vi "Mcp2210 Get Spi Config.vi"(6 "error in (no error)":errorcluster, 9 "handle":i32) -> (0 "error out":errorcluster, 2 "SPI Setting Out":T1 {"SPI Mode" items=["Mode 0", "Mode 1", "Mode 2", "Mode 3"]; "Baud Rate" format="%.0p"}, 3 "handle out":i32)   [LabVIEW 2015, in "mcp2210.lvlib"]
doc: "Get the SPI transfer settings for current (VM) configuration or for power-up\ndefault (NVRAM) SPI configuration.\nParameters:\nInputs:\n- void *handle - The pointer to the device handle. Cannot be NULL.\n- unsigned char cfgSelector - current/power-up chip setting selection. Valid values are:\n- MCP2210_VM_CONFIG: designates current chip setting (Volatile\nMemory)\n- MCP2210_NVRAM_CONFIG: designates power-up chip setting (NVRAM)\nOutputs:\n- unsigned int *pbaudRate - transfer speed. Cannot be NULL.\n- unsigned int *pidleCsVal - IDLE chip select value. Cannot be NULL.\nbit31 - - - - bit8 bit0\nx x ... x x CS8 CS7 CS6 CS5 CS4 CS3 CS2 CS1 CS0\n- unsigned int *pactiveCsVal - Active Chip Select Value. Cannot be NULL.\nbit31 - - - - bit8 bit0\nx x ... x x CS8 CS7 CS6 CS5 CS4 CS3 CS2 CS1 CS0\n- unsigned int *pCsToDataDly - Chip Select to Data Delay (quanta of 100 us)\n- 16-bit value => max value is (2^16-1).\n- Cannot be NULL.\n- unsigned int *pdataToCsDly - Last Data Byte to CS (de-asserted) Delay (quanta of 100 us)\n- 16-bit value => max value is (2^16)-1.\n- Cannot be NULL.\n- unsigned int *pdataToDataDly - Delay Between Subsequent Data Bytes (quanta of 100 us)\n- 16-bit value => max value is (2^16)-1.\n- Cannot be NULL.\n- unsigned int *ptxferSize - Bytes to Transfer per SPI Transaction.\n- 16-bit value => max value is (2^16)-1.\n- Cannot be NULL.\n- unsigned char *pspiMd - SPI Mode. Cannot be NULL.\nValid values are:\n- MCP2210_SPI_MODE0\n- MCP2210_SPI_MODE1\n- MCP2210_SPI_MODE2\n- MCP2210_SPI_MODE3\nReturns:\n- 0 for success: E_SUCCESS\n- negative error code: E_ERR_NULL, E_ERR_INVALID_HANDLE_VALUE\nE_ERR_UNKOWN_ERROR, E_ERR_INVALID_PARAMETER\nE_ERR_HID_TIMEOUT, E_ERR_HID_RW_FILEIO\nE_ERR_CMD_ECHO, E_ERR_CMD_FAILED\n\nMCP2210_DLL_UM_API int __stdcall Mcp2210_GetSpiConfig(void *handle, unsigned char cfgSelector, unsigned int *pbaudRate, unsigned int *pidleCsVal,\n unsigned int *pactiveCsVal, unsigned int *pCsToDataDly, unsigned int *pdataToCsDly,\n unsigned int *pdataToDataDly, unsigned int *ptxferSize, unsigned char *pspiMd);"
uses:
  <userlib>/mcp2210/mcp2210.lvlib
  <userlib>/mcp2210/mcp2210_dll_um_x86.dll
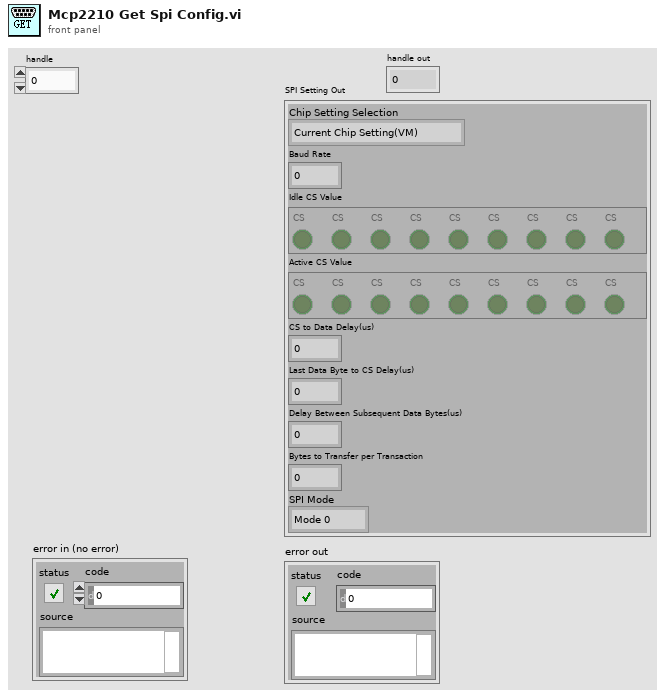
[diagram p1: front panel]
types:
  T1 = cluster{"Chip Setting Selection":enum8{"Current Chip Setting(VM)", "Power-up Chip Setting(NVRAM)"}, "Baud Rate":u32, "Idle CS Value":bool[], "Active CS Value":bool[], "CS to Data Delay(us)":u32, "Last Data Byte to CS Delay(us)":u32, "Delay Between Subsequent Data Bytes(us)":u32, "Bytes to Transfer per Transaction":u32, "SPI Mode":u8}
  T2 = cluster{"cfgSelector":u8, "pbaudRate":u32, "Boolean array":bool[], "Boolean array":bool[], u32, u32, u32, "ptxferSize":u32, u8}
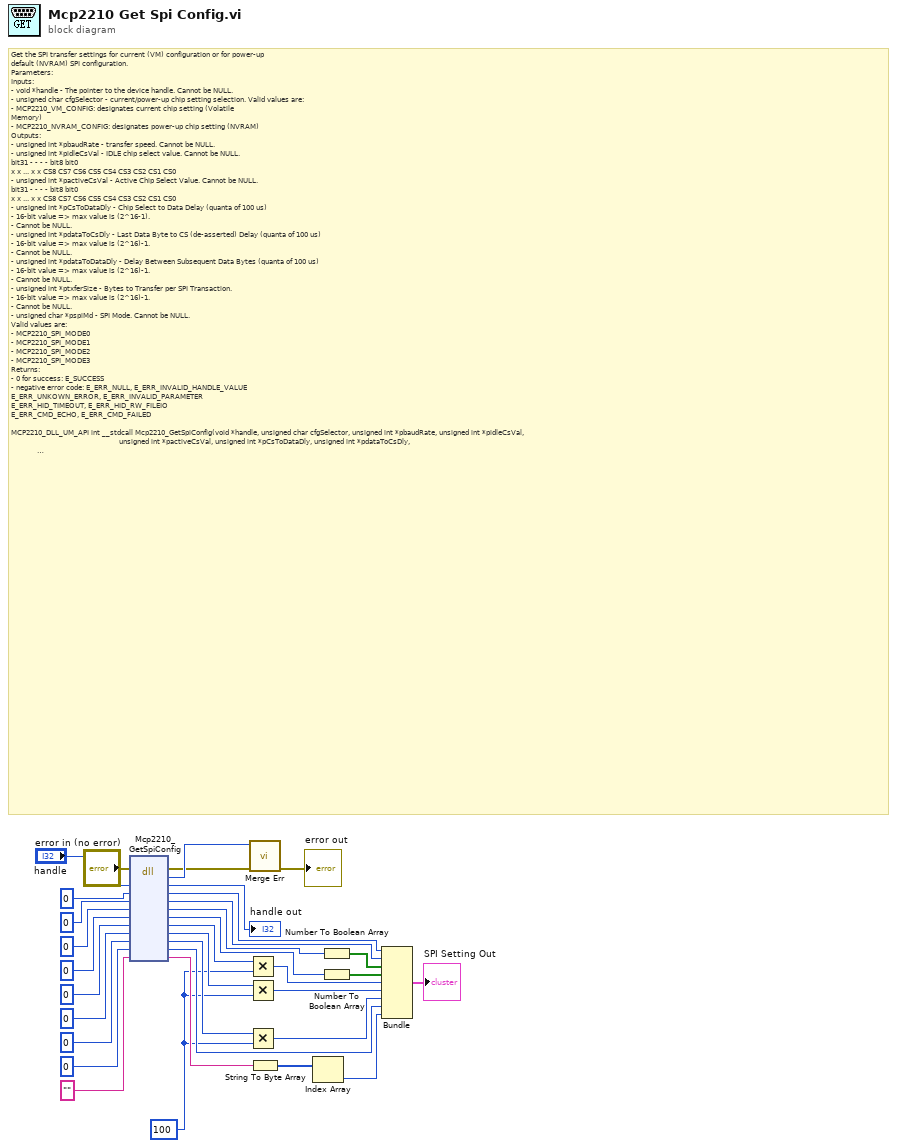
[diagram p0: block diagram]
diagram:
  w2 = u32 100 ("y")
  # "Get the SPI transfer settings for current (VM) configuration or for power-up\ndefault (NVRAM) SPI configuration.\nParameters:\nInputs:\n- void *handle - The pointer to the device handle. Cannot be NULL.\n- unsigned char cfgSelector - current/power-up chip setting selection. Valid values are:\n- MCP2210_VM_CONFIG: designates current chip setting (Volatile\nMemory)\n- MCP2210_NVRAM_CONFIG: designates power-up chip setting (NVRAM)\nOutputs:\n- unsigned int *pbaudRate - transfer speed. Cannot be NULL.\n- unsigned int *pidleCsVal - IDLE chip select value. Cannot be NULL.\nbit31 - - - - bit8 bit0\nx x ... x x CS8 CS7 CS6 CS5 CS4 CS3 CS2 CS1 CS0\n- unsigned int *pactiveCsVal - Active Chip Select Value. Cannot be NULL.\nbit31 - - - - bit8 bit0\nx x ... x x CS8 CS7 CS6 CS5 CS4 CS3 CS2 CS1 CS0\n- unsigned int *pCsToDataDly - Chip Select to Data Delay (quanta of 100 us)\n- 16-bit value => max value is (2^16-1).\n- Cannot be NULL.\n- unsigned int *pdataToCsDly - Last Data Byte to CS (de-asserted) Delay (quanta of 100 us)\n- 16-bit value => max value is (2^16)-1.\n- Cannot be NULL.\n- unsigned int *pdataToDataDly - Delay Between Subsequent Data Bytes (quanta of 100 us)\n- 16-bit value => max value is (2^16)-1.\n- Cannot be NULL.\n- unsigned int *ptxferSize - Bytes to Transfer per SPI Transaction.\n- 16-bit value => max value is (2^16)-1.\n- Cannot be NULL.\n- unsigned char *pspiMd - SPI Mode. Cannot be NULL.\nValid values are:\n- MCP2210_SPI_MODE0\n- MCP2210_SPI_MODE1\n- MCP2210_SPI_MODE2\n- MCP2210_SPI_MODE3\nReturns:\n- 0 for success: E_SUCCESS\n- negative error code: E_ERR_NULL, E_ERR_INVALID_HANDLE_VALUE\nE_ERR_UNKOWN_ERROR, E_ERR_INVALID_PARAMETER\nE_ERR_HID_TIMEOUT, E_ERR_HID_RW_FILEIO\nE_ERR_CMD_ECHO, E_ERR_CMD_FAILED\n\nMCP2210_DLL_UM_API int __stdcall Mcp2210_GetSpiConfig(void *handle, unsigned char cfgSelector, unsigned int *pbaudRate, unsigned int *pidleCsVal,\n                                                      unsigned int *pactiveCsVal, unsigned int *pCsToDataDly, unsigned int *pdataToCsDly,\n                                                      unsigned int *pdataToDataDly, unsigned int *ptxferSize, unsigned char *pspiMd);"
  n1 = dll-call lib="D:/LabVIEW 2015/user.lib/mcp2210/mcp2210_dll_um_x86.*" fn="Mcp2210_GetSpiConfig"(error in="error in (no error)", "handle"="handle", "cfgSelector"=u8 0, "pbaudRate"=u32 0, "pidleCsVal"=u32 0, "pactiveCsVal"=u32 0, "pCsToDataDly"=u32 0, "pdataToCsDly"=u32 0, "pdataToDataDly"=u32 0, "ptxferSize"=u32 0, "pspiMd"="") -> (error out=w12:errorcluster, "return type"=w13:i32, "handle"=→"handle out":i32, "cfgSelector"=w14:u8, "pbaudRate"=w11:u32, "pidleCsVal"=w10:u32, "pactiveCsVal"=w9:u32, "pCsToDataDly"=w8:u32, "pdataToCsDly"=w7:u32, "pdataToDataDly"=w6:u32, "ptxferSize"=w4:u32, "pspiMd"=w5:string)  [unwired: 2 in, 1 out]
  n2 = Multiply(x=w8, y=w2) -> (x*y=w20:u32)
  n3 = Multiply(x=w7, y=w2) -> (x*y=w19:u32)
  n4 = Multiply(x=w6, y=w2) -> (x*y=w18:u32)
  n5 = call <userlib>:"Merge Err.vi"("error in (no error)"=w12, "return type"=w13) -> ("error out"=→"error out":errorcluster)  [unwired: 9 in]
  n6 = String To Byte Array(string=w5) -> (unsigned byte array=w17:u8[])
  n7 = Index Array(array=w17) -> (element=w16:u8)  [unwired: 1 in]
  n8 = Number To Boolean Array(number=w10) -> (Boolean array=w22:bool[])
  n9 = Number To Boolean Array(number=w9) -> (Boolean array=w21:bool[])
  n10 = Bundle("cfgSelector"=w14, "pbaudRate"=w11, "Boolean array"=w22, "Boolean array"=w21, w20, w19, w18, "ptxferSize"=w4, w16) -> (→"SPI Setting Out":T2)  [unwired: 1 in]
